vi "InitializeJSONFile.vi"() -> (1 "Path":path, 4 "error out":errorcluster)   [LabVIEW 2018]
uses:
  Global Variables.vi
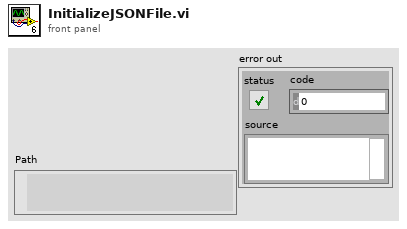
[diagram p1: front panel]
types:
  T1 = enum16{"open", "replace", "create", "open or create", "replace or create", "replace or create with confirmation"}
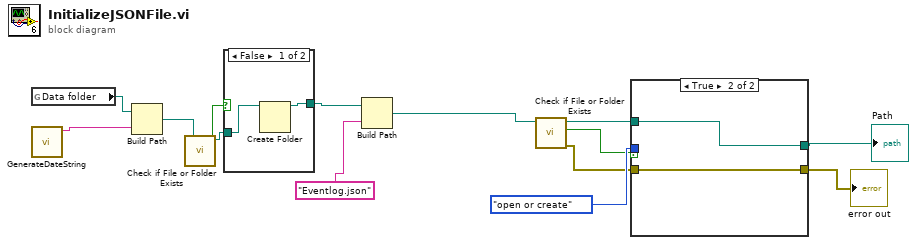
[diagram p0: block diagram]
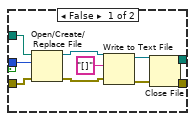
[diagram p2: hidden frame]
diagram:
  n1 = global read "Global Variables.vi" "Data folder"() -> (w7:path)
  n2 = call "GenerateDateString.vi"() -> ("String"=w8:string)  [unwired: 11 in]
  n3 = Build Path(base path=w7, name or relative path=w8) -> (appended path=w11:path)
  n4 = call <vilib>:"Check if File or Folder Exists.vi"("path"=w11) -> ("file or folder exists?"=w9:bool, "dup path"=w10:path)  [unwired: 8 in, 1 out]
  n5 = case shown="False" w9 {
    tunnel: w10 -> [w16 w17]
    tunnel: [w15 w17] -> w12
    frame False {
      n6 = Create Folder(path (use dialog)=w16) -> (created path=w15:path)  [unwired: 2 in, 2 out]
    }
    frame True {
    }
  }
  n7 = Build Path(base path=w12, name or relative path="Eventlog.json" ("string")) -> (appended path=w4:path)
  n8 = call <vilib>:"Check if File or Folder Exists.vi"("path"=w4) -> ("error out"=w2:errorcluster, "file or folder exists?"=w1:bool, "dup path"=w3:path)  [unwired: 8 in]
  n9 = case shown="True" w1 {
    tunnel: T1."open or create" ("operation (0:open)") -> [w27 _]
    tunnel: [w21 w28] -> w6
    tunnel: [w20 w29] -> w5
    tunnel: w3 -> [w19 w29]
    tunnel: w2 -> [w18 w28]
    frame False {
      n10 = Open/Create/Replace File(file path (use dialog)=w19, error in=w18, operation (0:open)=w27) -> (refnum out=w25:refnum<file>, error out=w24:errorcluster)  [unwired: 3 in, 1 out]
      n11 = Write to Text File(file (use dialog)=w25, text="[]", error in=w24) -> (refnum out=w22:refnum<file>, error out=w23:errorcluster)  [unwired: 1 in, 1 out]
      n12 = Close File(refnum=w22, error in=w23) -> (path=w20:path, error out=w21:errorcluster)
    }
    frame True {
    }
  }
  "Path" <- w5
  "error out" <- w6
